vi "2D Cartesian Coordinate Rotation (Array).vi"(9 "theta":dbl, 10 "Y":dbl[](array[numeric]), 11 "X":dbl[](array[numeric])) -> (0 "error":i32, 2 "Y Out":dbl[](array[numeric]), 3 "X Out":dbl[](array[numeric]))   [LabVIEW 2017, in "NI_AALPro.lvlib"]
doc: "Rotates a two-dimensional Cartesian coordinate system in the counterclockwise direction. Wire data to the <B>X</B> input to determine the polymorphic instance to use or manually select the instance."
uses:
  NI_AALPro.lvlib
  lvanlys.dll
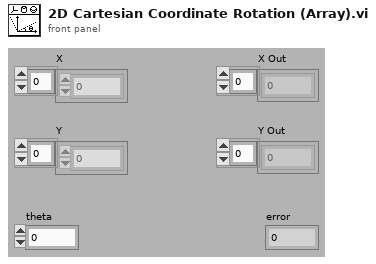
[diagram p1: front panel]
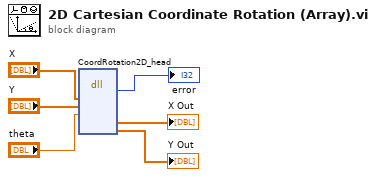
[diagram p0: block diagram]
diagram:
  n1 = dll-call lib="C:/Program Files/National Instruments/LabVIEW 2017/resource/lvanlys.*" fn="CoordRotation2D_head"("X"="X", "Y"="Y", "theta"="theta") -> (→"error":i32, "Xout"=→"X Out":dbl[], "Yout"=→"Y Out":dbl[])  [unwired: 8 in, 2 out]
